vi "CarWashClientMain.vi"() -> ()   [LabVIEW 2024]
uses:
  CarWashState.ctl
  Deluxeglobal.vi
panel:
  out "VehicleOut":bool
  out "AirDry":bool
  out "CW Rinse":bool
  out "MHPWash":bool
  out "SoapApp":bool
  out "UB Wash":bool
  in  "Car Wash Simulation Switches":T1
  out "Wash Selection":string
  in  "stop":bool
  in  "Economy":bool
  in  "Deluxe":bool
  out "error out":errorcluster
  in  "error in (no error)":errorcluster
  # "Car Wash Indicators"
  # "Purchase Selection"
  # "Deluxe Wash"
  # "Under Body Wash"
  # "Economy Wash"
  # "Soap Application"
  # "Main High Pressure Wash"
  # "Clear Water Rinse"
  # "Air Dry"
  # "Vehicle Out of Position"
  # "Under Body\nPosition Wash\nSwitch"
  # "Air Dry\nSwitch"
  # "Main Wash\nPosition \nSwitch"
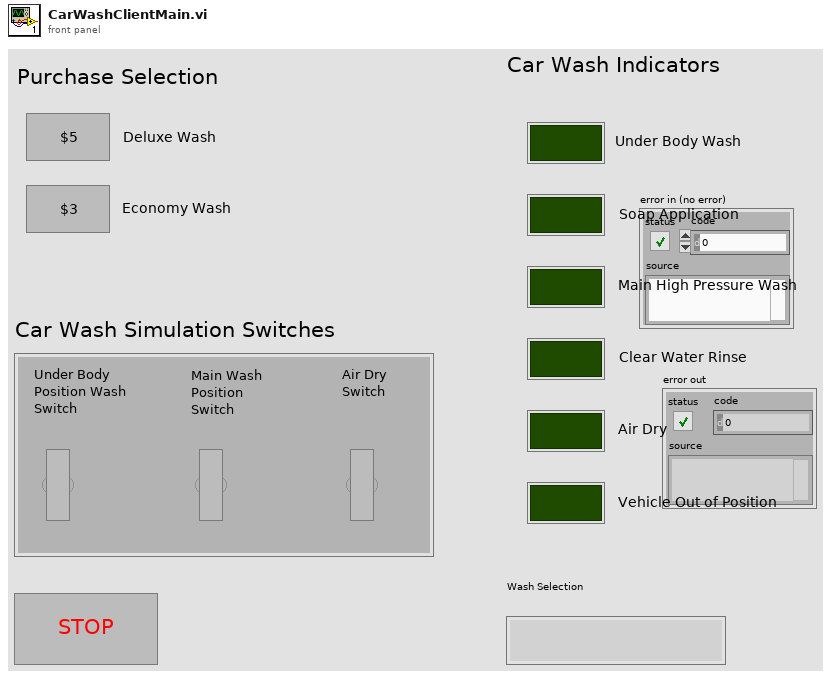
[diagram p1: front panel]
types:
  T1 = cluster{"UB Switch":bool, "MW Switch":bool, "ADSwitch":bool}
  T2 = typedef "CarWashState.ctl" = enum16{"Initialization", "Select Wash", "UnderBody Wash", "Soap Application", "Main High pressure Wash", "Clear Water Rinse", "Air Dry", "DataTransmission", "Clean up", "stop"}
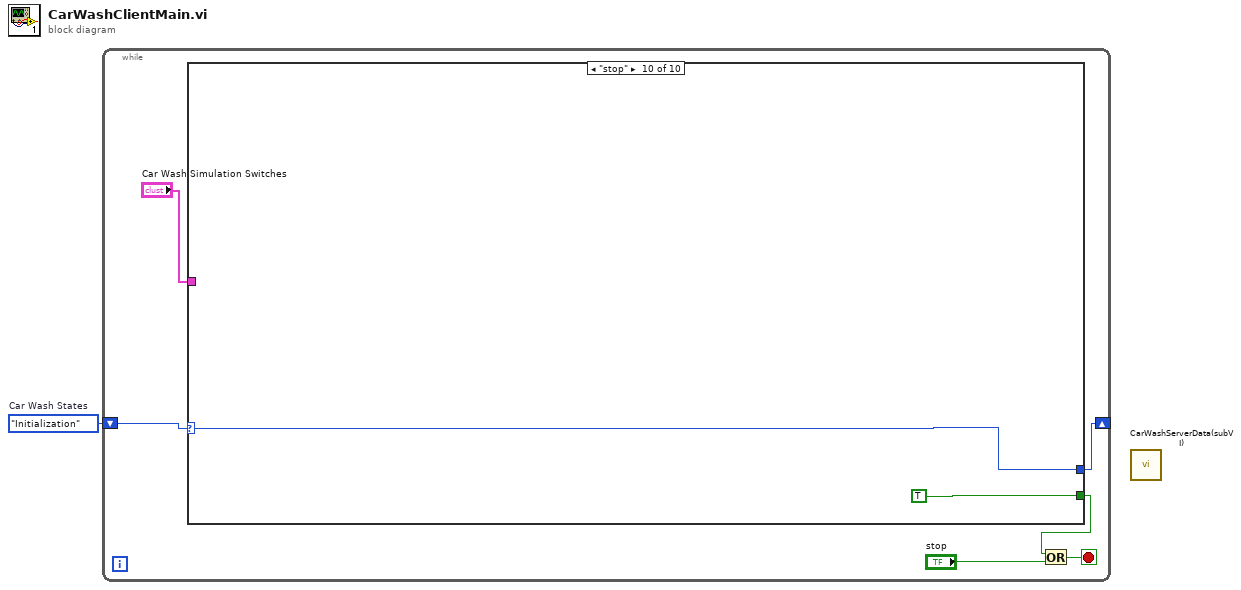
[diagram p0: block diagram]
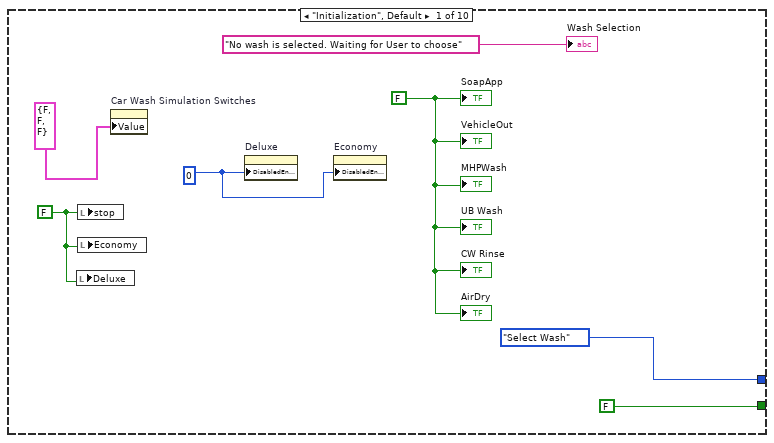
[diagram p2: hidden frame]
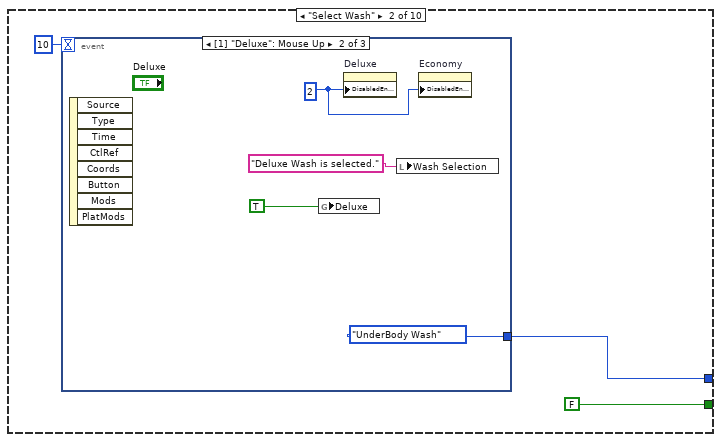
[diagram p3: hidden frame]
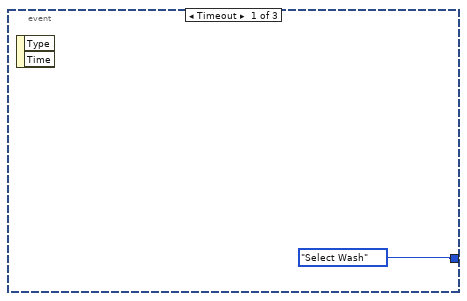
[diagram p4: hidden frame]
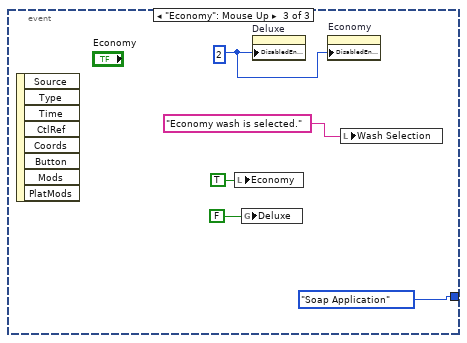
[diagram p5: hidden frame]
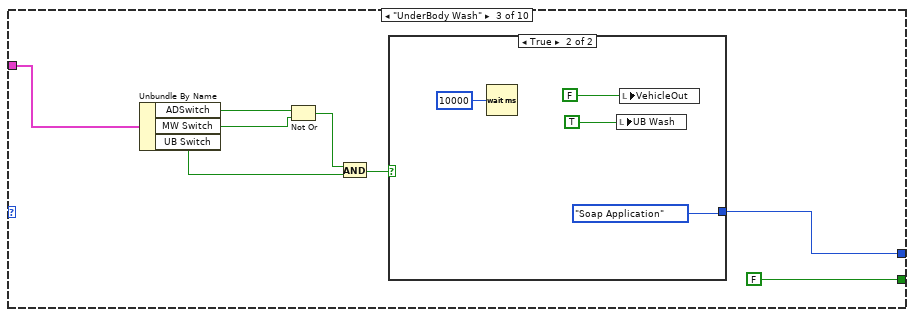
[diagram p6: hidden frame]
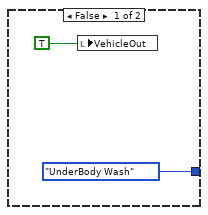
[diagram p7: hidden frame]
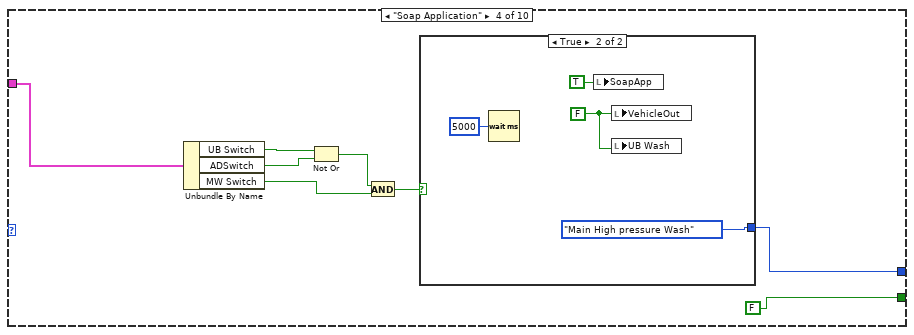
[diagram p8: hidden frame]
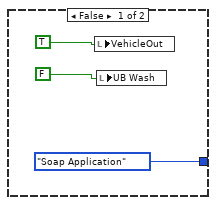
[diagram p9: hidden frame]
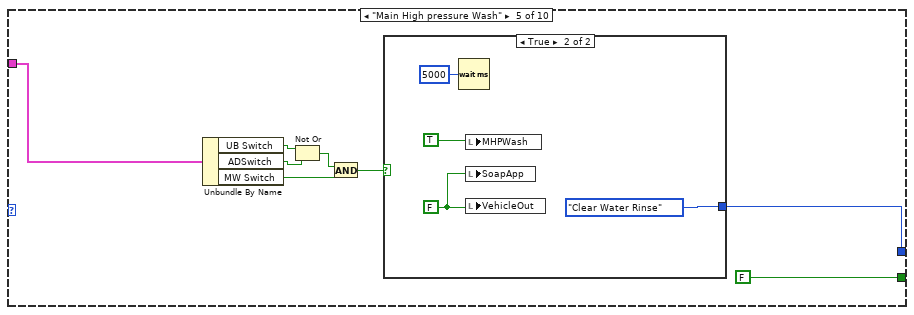
[diagram p10: hidden frame]
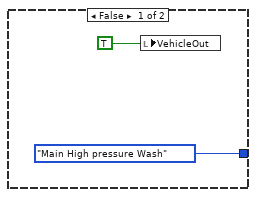
[diagram p11: hidden frame]
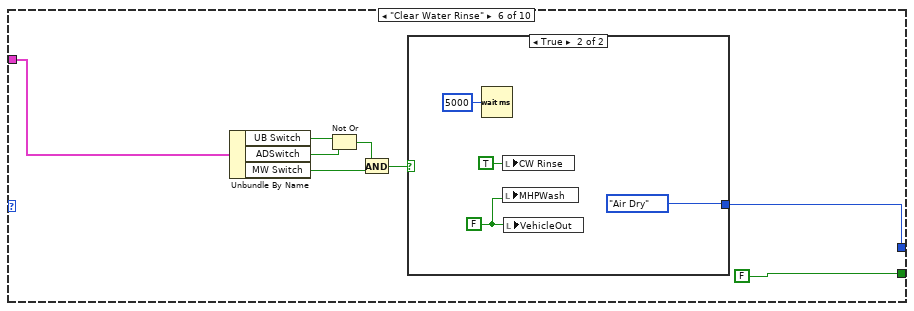
[diagram p12: hidden frame]
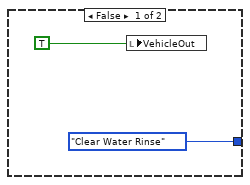
[diagram p13: hidden frame]
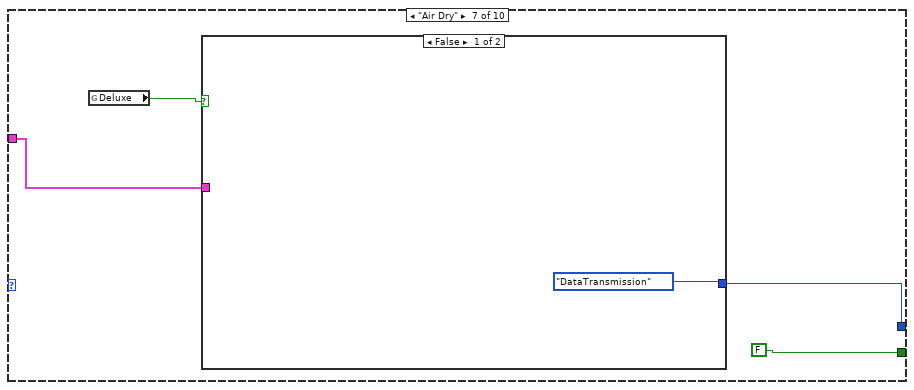
[diagram p14: hidden frame]
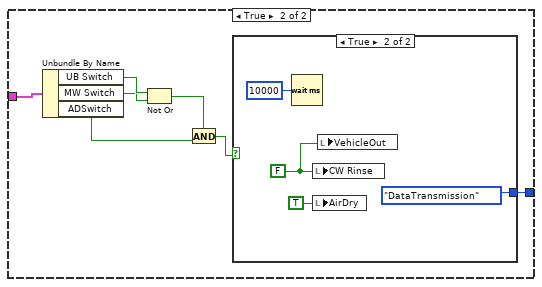
[diagram p15: hidden frame]
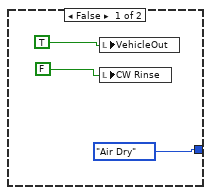
[diagram p16: hidden frame]
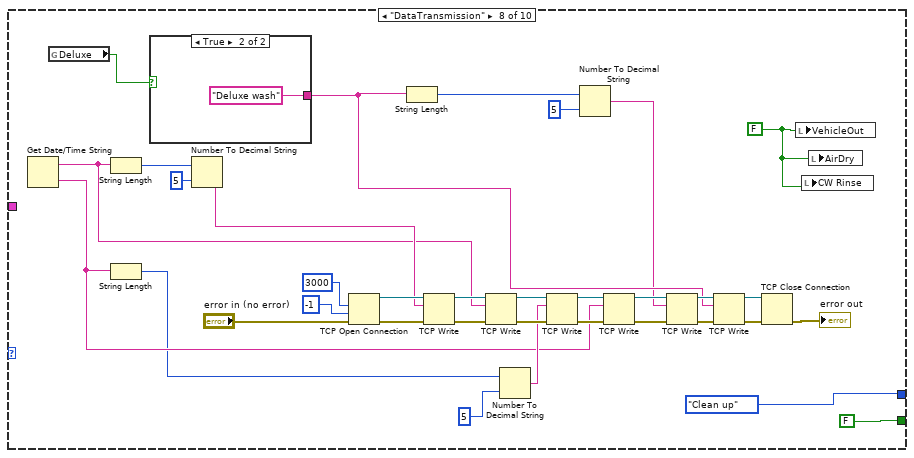
[diagram p17: hidden frame]
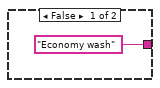
[diagram p18: hidden frame]
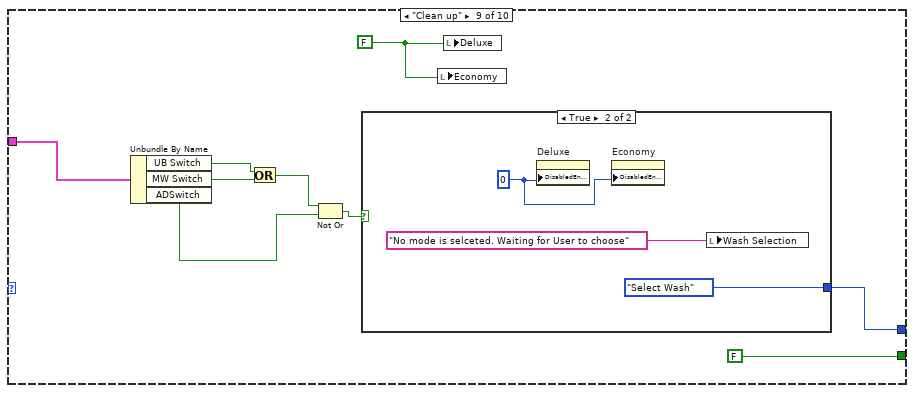
[diagram p19: hidden frame]
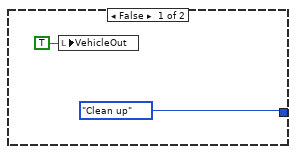
[diagram p20: hidden frame]
diagram:
  w1 = CarWashState."Initialization"  # Car Wash States
  n1 = while {
    shift-right: [w2] -> _
    shift-left: w1 -> [w3]
    stop <- w4 stop-if-true
    n2 = case shown="\"stop\"" w3 {
      selector: w3 -> [_ _ _ _ _ _ _ _ _ w154]
      tunnel: "Car Wash Simulation Switches" -> [_ _ w35 w49 w64 w78 w88 _ w146 _]
      tunnel: [FALSE FALSE FALSE FALSE FALSE FALSE FALSE FALSE FALSE TRUE] -> w6
      tunnel: [CarWashState."Select Wash" w15 w28 w42 w57 w71 w85 CarWashState."Clean up" ("Car Wash States") w147 w154] -> w2
      frame "Initialization", Default {
        w8 = FALSE ("SoapApp")
        w13 = 0
        w11 = FALSE
        n3 = local write "Deluxe"(w11) -> ()
        n4 = local write "stop"(w11) -> ()
        n5 = local write "Economy"(w11) -> ()
        n6 = property on="Car Wash Simulation Switches" class="Clust (strict)"("Value"=T1 {"UB Switch"=FALSE, "MW Switch"=FALSE, "ADSwitch"=FALSE} ("Car Wash Simulation Switches")) -> ()  [unwired: 2 in, 2 out]
        n7 = property on="Deluxe" class="Bool (strict)"("DisabledEnum"=w13) -> ()  [unwired: 2 in, 2 out]
        n8 = property on="Economy" class="Bool (strict)"("DisabledEnum"=w13) -> ()  [unwired: 2 in, 2 out]
        "Wash Selection" <- "No wash is selected. Waiting for User to choose" ("Wash Selection")
        "AirDry" <- w8
        "VehicleOut" <- w8
        "SoapApp" <- w8
        "MHPWash" <- w8
        "CW Rinse" <- w8
        "UB Wash" <- w8
      }
      frame "Select Wash" {
        n9 = event shown="[1] \"Deluxe\": Mouse Up" {
          selector: _ -> [_ _ _]
          dyn-events: _ -> [_ _ _]
          timeout: 10 -> [_ _ _]
          tunnel: [CarWashState."Select Wash" CarWashState."UnderBody Wash" CarWashState."Soap Application"] -> w15
          event Timeout {
            n10 = event-data() -> ()  [unwired: 1 in, 2 out]
          }
          event "Deluxe": Mouse Up {
            w21 = 2
            n11 = event-data() -> ()  [unwired: 1 in, 8 out]
            n12 = global write "Deluxeglobal.vi" "Deluxe"(TRUE ("Deluxe")) -> ()
            n13 = property on="Deluxe" class="Bool (strict)"("DisabledEnum"=w21) -> ()  [unwired: 2 in, 2 out]
            n14 = local write "Wash Selection"("Deluxe Wash is selected." ("Wash Selection")) -> ()
            n15 = property on="Economy" class="Bool (strict)"("DisabledEnum"=w21) -> ()  [unwired: 2 in, 2 out]
          }
          event "Economy": Mouse Up {
            w26 = 2
            n16 = event-data() -> ()  [unwired: 1 in, 8 out]
            n17 = local write "Economy"(TRUE ("Economy")) -> ()
            n18 = global write "Deluxeglobal.vi" "Deluxe"(FALSE ("Economy")) -> ()
            n19 = property on="Deluxe" class="Bool (strict)"("DisabledEnum"=w26) -> ()  [unwired: 2 in, 2 out]
            n20 = property on="Economy" class="Bool (strict)"("DisabledEnum"=w26) -> ()  [unwired: 2 in, 2 out]
            n21 = local write "Wash Selection"("Economy wash is selected." ("Wash Selection")) -> ()
          }
        }
      }
      frame "UnderBody Wash" {
        n22 = Unbundle By Name(w35) -> ("ADSwitch"=w34:bool, "MW Switch"=w33:bool, "UB Switch"=w31:bool)
        n23 = Not Or(1:w33, 2:w34) -> (0:w32:bool)
        n24 = And(x=w32, y=w31) -> (x .and. y?=w29:bool)
        n25 = case shown="True" w29 {
          tunnel: [CarWashState."UnderBody Wash" CarWashState."Soap Application" ("Car Wash States")] -> w28
          frame False {
            n26 = local write "VehicleOut"(TRUE) -> ()
          }
          frame True {
            n27 = Wait (ms)(milliseconds to wait=u32 10000) -> ()  [unwired: 1 out]
            n28 = local write "UB Wash"(TRUE) -> ()
            n29 = local write "VehicleOut"(FALSE) -> ()
          }
        }
      }
      frame "Soap Application" {
        n30 = Unbundle By Name(w49) -> ("UB Switch"=w48:bool, "ADSwitch"=w47:bool, "MW Switch"=w45:bool)
        n31 = Not Or(1:w47, 2:w48) -> (0:w46:bool)
        n32 = And(x=w46, y=w45) -> (x .and. y?=w44:bool)
        n33 = case shown="True" w44 {
          tunnel: [CarWashState."Soap Application" CarWashState."Main High pressure Wash" ("Car Wash States")] -> w42
          frame False {
            n34 = local write "VehicleOut"(TRUE) -> ()
            n35 = local write "UB Wash"(FALSE) -> ()
          }
          frame True {
            w53 = FALSE ("VehicleOut")
            n36 = Wait (ms)(milliseconds to wait=u32 5000) -> ()  [unwired: 1 out]
            n37 = local write "SoapApp"(TRUE ("SoapApp")) -> ()
            n38 = local write "VehicleOut"(w53) -> ()
            n39 = local write "UB Wash"(w53) -> ()
          }
        }
      }
      frame "Main High pressure Wash" {
        n40 = Unbundle By Name(w64) -> ("UB Switch"=w62:bool, "ADSwitch"=w61:bool, "MW Switch"=w59:bool)
        n41 = Not Or(1:w61, 2:w62) -> (0:w60:bool)
        n42 = And(x=w60, y=w59) -> (x .and. y?=w58:bool)
        n43 = case shown="True" w58 {
          tunnel: [CarWashState."Main High pressure Wash" CarWashState."Clear Water Rinse" ("Car Wash States")] -> w57
          frame False {
            n44 = local write "VehicleOut"(TRUE) -> ()
          }
          frame True {
            w67 = FALSE ("VehicleOut")
            n45 = Wait (ms)(milliseconds to wait=u32 5000) -> ()  [unwired: 1 out]
            n46 = local write "MHPWash"(TRUE ("MHPWash")) -> ()
            n47 = local write "SoapApp"(w67) -> ()
            n48 = local write "VehicleOut"(w67) -> ()
          }
        }
      }
      frame "Clear Water Rinse" {
        n49 = Unbundle By Name(w78) -> ("UB Switch"=w76:bool, "ADSwitch"=w75:bool, "MW Switch"=w73:bool)
        n50 = Not Or(1:w75, 2:w76) -> (0:w74:bool)
        n51 = And(x=w74, y=w73) -> (x .and. y?=w72:bool)
        n52 = case shown="True" w72 {
          tunnel: [CarWashState."Clear Water Rinse" CarWashState."Air Dry" ("Car Wash States")] -> w71
          frame False {
            n53 = local write "VehicleOut"(TRUE) -> ()
          }
          frame True {
            w81 = FALSE ("VehicleOut")
            n54 = Wait (ms)(milliseconds to wait=u32 5000) -> ()  [unwired: 1 out]
            n55 = local write "CW Rinse"(TRUE ("CW Rinse")) -> ()
            n56 = local write "MHPWash"(w81) -> ()
            n57 = local write "VehicleOut"(w81) -> ()
          }
        }
      }
      frame "Air Dry" {
        n58 = global read "Deluxeglobal.vi" "Deluxe"() -> (w86:bool)
        n59 = case shown="False" w86 {
          tunnel: w88 -> [_ w96]
          tunnel: [CarWashState."DataTransmission" ("Car Wash States") w90] -> w85
          frame False {
          }
          frame True {
            n60 = Unbundle By Name(w96) -> ("UB Switch"=w95:bool, "MW Switch"=w94:bool, "ADSwitch"=w92:bool)
            n61 = Not Or(1:w94, 2:w95) -> (0:w93:bool)
            n62 = And(x=w93, y=w92) -> (x .and. y?=w91:bool)
            n63 = case shown="True" w91 {
              tunnel: [CarWashState."Air Dry" CarWashState."DataTransmission" ("Car Wash States")] -> w90
              frame False {
                n64 = local write "VehicleOut"(TRUE) -> ()
                n65 = local write "CW Rinse"(FALSE) -> ()
              }
              frame True {
                w100 = FALSE ("CW Rinse")
                n66 = Wait (ms)(milliseconds to wait=u32 10000) -> ()  [unwired: 1 out]
                n67 = local write "CW Rinse"(w100) -> ()
                n68 = local write "AirDry"(TRUE ("AirDry")) -> ()
                n69 = local write "VehicleOut"(w100) -> ()
              }
            }
          }
        }
      }
      frame "DataTransmission" {
        w107 = FALSE
        n70 = Get Date/Time String() -> (date string=w113:string, time string=w110:string)  [unwired: 3 in]
        n71 = global read "Deluxeglobal.vi" "Deluxe"() -> (w137:bool)
        n72 = String Length(string=w113) -> (length=w134:i32)
        n73 = String Length(string=w110) -> (length=w109:i32)
        n74 = case shown="True" w137 {
          tunnel: ["Economy wash" "Deluxe wash"] -> w112
          frame False {
          }
          frame True {
          }
        }
        n75 = Number To Decimal String(number=w134, width (-)=i16 5) -> (decimal integer string=w114:string)
        n76 = TCP Open Connection(remote port or service name=u16 3000, timeout ms (60000)=-1, error in (no error)="error in (no error)") -> (connection ID=w132:refnum<k5>, error out=w131:errorcluster)  [unwired: 2 in]
        n77 = String Length(string=w112) -> (length=w136:i32)
        n78 = TCP Write(connection ID=w132, data in=w114, error in (no error)=w131) -> (connection ID out=w130:refnum<k5>, error out=w129:errorcluster)  [unwired: 1 in, 1 out]
        n79 = TCP Write(connection ID=w130, data in=w113, error in (no error)=w129) -> (connection ID out=w128:refnum<k5>, error out=w127:errorcluster)  [unwired: 1 in, 1 out]
        n80 = Number To Decimal String(number=w109, width (-)=i16 5) -> (decimal integer string=w118:string)
        n81 = TCP Write(connection ID=w128, data in=w118, error in (no error)=w127) -> (connection ID out=w126:refnum<k5>, error out=w125:errorcluster)  [unwired: 1 in, 1 out]
        n82 = Number To Decimal String(number=w136, width (-)=i16 5) -> (decimal integer string=w111:string)
        n83 = TCP Write(connection ID=w126, data in=w110, error in (no error)=w125) -> (connection ID out=w120:refnum<k5>, error out=w119:errorcluster)  [unwired: 1 in, 1 out]
        n84 = TCP Write(connection ID=w120, data in=w111, error in (no error)=w119) -> (connection ID out=w124:refnum<k5>, error out=w123:errorcluster)  [unwired: 1 in, 1 out]
        n85 = TCP Write(connection ID=w124, data in=w112, error in (no error)=w123) -> (connection ID out=w122:refnum<k5>, error out=w121:errorcluster)  [unwired: 1 in, 1 out]
        n86 = TCP Close Connection(connection ID=w122, error in (no error)=w121) -> (error out=→"error out":errorcluster)  [unwired: 1 in, 1 out]
        n87 = local write "VehicleOut"(w107) -> ()
        n88 = local write "CW Rinse"(w107) -> ()
        n89 = local write "AirDry"(w107) -> ()
      }
      frame "Clean up" {
        w140 = FALSE
        n90 = Unbundle By Name(w146) -> ("UB Switch"=w145:bool, "MW Switch"=w144:bool, "ADSwitch"=w143:bool)
        n91 = Or(x=w145, y=w144) -> (x .or. y?=w142:bool)
        n92 = Not Or(1:w143, 2:w142) -> (0:w141:bool)
        n93 = case shown="True" w141 {
          tunnel: [CarWashState."Clean up" ("Car Wash States") CarWashState."Select Wash"] -> w147
          frame False {
            n94 = local write "VehicleOut"(TRUE ("VehicleOut")) -> ()
          }
          frame True {
            w153 = 0
            n95 = property on="Deluxe" class="Bool (strict)"("DisabledEnum"=w153) -> ()  [unwired: 2 in, 2 out]
            n96 = property on="Economy" class="Bool (strict)"("DisabledEnum"=w153) -> ()  [unwired: 2 in, 2 out]
            n97 = local write "Wash Selection"("No mode is selceted. Waiting for User to choose" ("Wash Selection")) -> ()
          }
        }
        n98 = local write "Economy"(w140) -> ()
        n99 = local write "Deluxe"(w140) -> ()
      }
      frame "stop" {
      }
    }
    n100 = Or(x=w6, y="stop") -> (x .or. y?=w4:bool)
  }
  n101 = call "CarWashServerData(subVI).vi"() -> ()  [unwired: 9 in, 3 out]
